vi "Test4.vi"() -> ()   [LabVIEW 2024]
uses:
  PID Controller/PID Controller/PID Controller.lvclass
  PID Controller/PID Controller Messages/Set Loop Period Msg/Set Loop Period Msg.lvclass/Set Loop Period Msg.ctl
  <vilib>/ActorFramework/Message Enqueuer/Message Enqueuer.lvclass/Message Enqueuer.ctl
  <vilib>/ActorFramework/Message Enqueuer/Enqueue.vi
  PID Controller/PID Controller Messages/Set Loop Period Msg/Set Loop Period Msg.lvclass
  <vilib>/ActorFramework/Stop Msg/Stop Msg.lvclass
  <vilib>/ActorFramework/Message Priority Queue/Priority Enqueue.vi
  <vilib>/addons/control/pid/pid.llb/PID (DBL).vi
  <vilib>/ActorFramework/Actor/Actor.lvclass
  <vilib>/addons/control/pid/NI_PID_pid.lvlib
panel:
  in  "stop":bool
  out "Waveform Chart":dbl(graph)
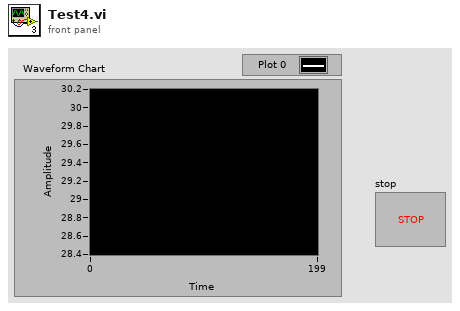
[diagram p1: front panel]
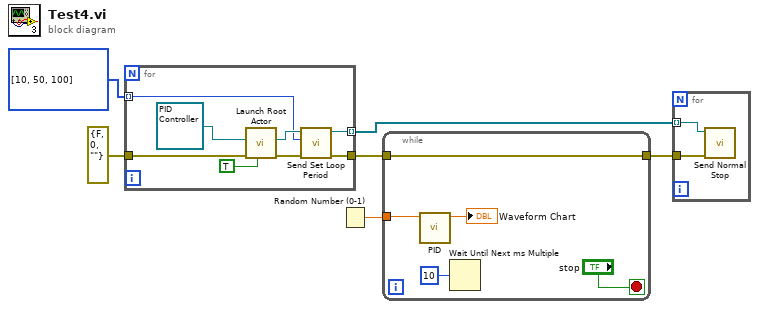
[diagram p0: block diagram]
diagram:
  n1 = for {
    tunnel: [w11] -> w3
    tunnel: errorcluster {"status"=FALSE, "code"=0, "source"=""} ("error in (no error)") -> [w10]
    tunnel: [w9] -> w5 mode=indexing
    tunnel: u32[] [10, 50, 100] -> [w7] mode=indexing
    n2 = call <vilib>:"Launch Root Actor.vi"("Open Actor Core front panel? (F)"=TRUE, "error in (no error)"=w10, "Actor"=refnum<class "PID Controller.lvclass"> refnum ("PID Controller.lvlib:PID Controller.lvclass")) -> ("error out"=w12:errorcluster, "Actor's Enqueuer"=w13:refnum<class "Message Enqueuer.lvclass">)  [unwired: 7 in]
    n3 = call "Send Set Loop Period.vi"("error in (no error)"=w12, "loop period"=w7, "Message Enqueuer"=w13) -> ("error out"=w11:errorcluster, "Message Enqueuer out"=w9:refnum<class "Message Enqueuer.lvclass">)  [unwired: 7 in]
  }
  n4 = Random Number (0-1)() -> (number: 0 to 1=w1:dbl)
  n5 = while {
    tunnel: [w18] -> w4
    tunnel: w3 -> [w18]
    tunnel: w1 -> [w15]
    stop <- "stop" stop-if-true
    n6 = call-poly <vilib>:"PID.vi"("setpoint"=w15) -> ("output"=→"Waveform Chart":dbl)  [unwired: 9 in, 1 out]
    n7 = Wait Until Next ms Multiple(millisecond multiple=u32 10) -> ()  [unwired: 1 out]
  }
  n8 = for {
    tunnel: w5 -> [w21] mode=indexing
    tunnel: w4 -> [w20]
    n9 = call <vilib>:"Send Normal Stop.vi"("error in (no error)"=w20, "Message Enqueuer"=w21) -> ()  [unwired: 9 in, 1 out]
  }
